vi "CosinusFunctionGraph.vi"() -> ()   [LabVIEW 2011]
panel:
  out "Waveform Graph":cluster{dbl, dbl, dbl[]}(graph)
  # "334AB ALEXANDRESCU Anda\nPanoul frontal pentru graficul functiei cosinus"
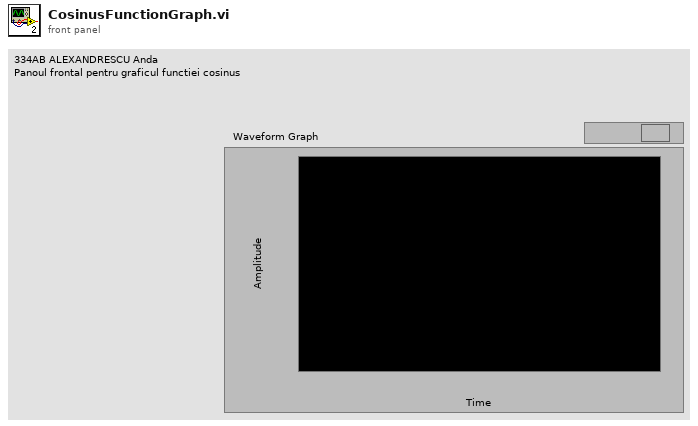
[diagram p1: front panel]
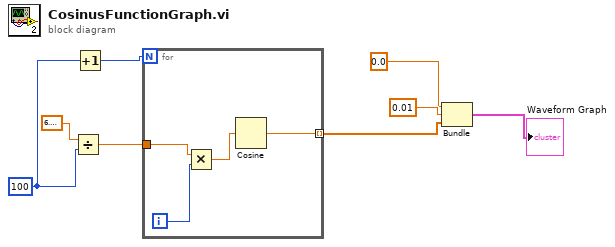
[diagram p0: block diagram]
diagram:
  w3 = 100
  n1 = Divide(x=6.283185307179586, y=w3) -> (x/y=w4:dbl)
  n2 = Increment(x=w3) -> (x+1=w2:i32)
  n3 = for {
    N: w2 -> [_]
    tunnel: [w11] -> w5 mode=indexing
    tunnel: w4 -> [w10]
    i -> [w9]
    n4 = Multiply(x=w10, y=w9) -> (x*y=w12:dbl)
    n5 = Cosine(x=w12) -> (cos(x)=w11:dbl)
  }
  n6 = Bundle(0.0, 0.01, w5) -> (→"Waveform Graph":cluster{dbl, dbl, dbl[]})  [unwired: 1 in]
